vi "Communication.vi"(8 "Error In":errorcluster, 10 "Command":string, 11 "connection ID":refnum<k5>) -> (0 "Error Out":errorcluster, 2 "Data out":string, 3 "connection ID out":refnum<k5>)   [LabVIEW 2019, in "TCP2Foxconn.lvlib"]
uses:
  TCP2Foxconn.lvlib
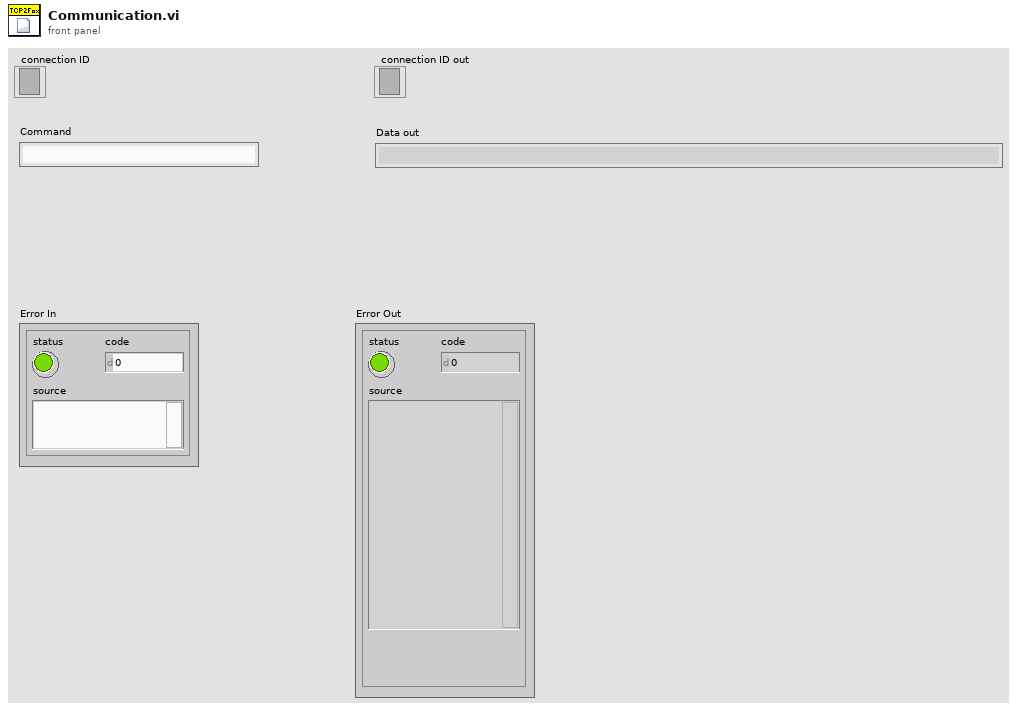
[diagram p1: front panel]
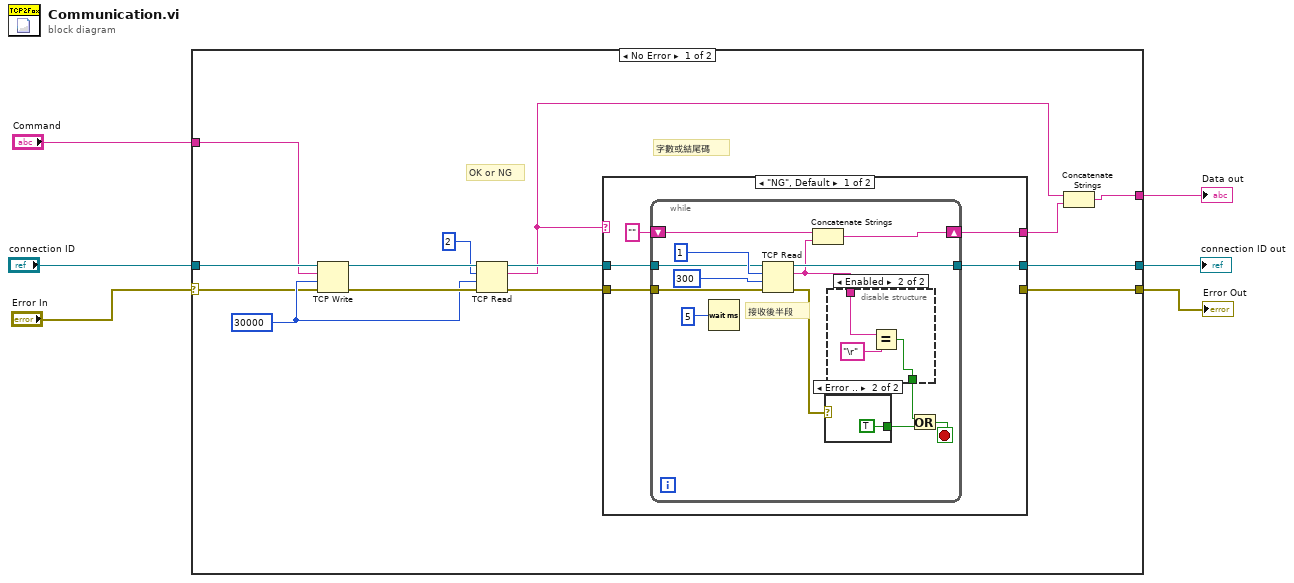
[diagram p0: block diagram]
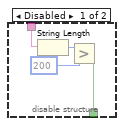
[diagram p2: hidden frame]
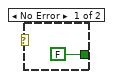
[diagram p3: hidden frame]
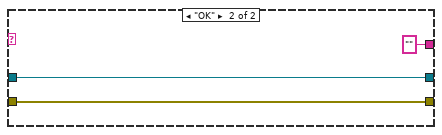
[diagram p4: hidden frame]
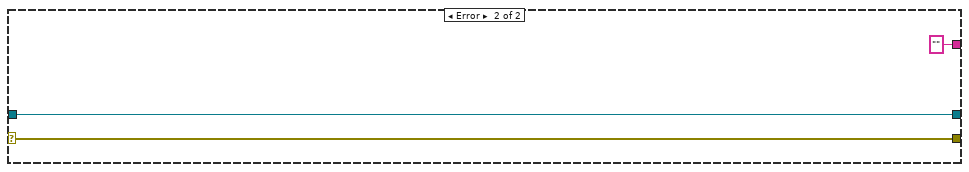
[diagram p5: hidden frame]
diagram:
  n1 = case shown="No Error" "Error In" {
    selector: "Error In" -> [w13 w52]
    tunnel: [w10 w52] -> w5
    tunnel: "connection ID" -> [w18 w53]
    tunnel: [w11 w53] -> w3
    tunnel: "Command" -> [w12 _]
    tunnel: [w7 "" ("data out")] -> w1
    frame No Error {
      w14 = 30000 ("timeout ms (25000)")
      # "字數或結尾碼"
      # "OK or NG"
      n2 = TCP Write(connection ID=w18, data in=w12, error in (no error)=w13, 9:w14) -> (connection ID out=w20:refnum<k5>, error out=w19:errorcluster)  [unwired: 1 out]
      n3 = TCP Read(connection ID=w20, bytes to read=2, error in (no error)=w19, 9:w14) -> (connection ID out=w15:refnum<k5>, data out=w9:string, error out=w16:errorcluster)  [unwired: 1 in]
      n4 = case shown="\"NG\", Default" w9 {
        tunnel: w16 -> [w24 w49]
        tunnel: w15 -> [w25 w50]
        tunnel: [_ w49] -> w10
        tunnel: [w22 w50] -> w11
        tunnel: [w21 ""] -> w8
        frame "NG", Default {
          n5 = while {
            tunnel: w25 -> [w36]
            tunnel: w24 -> [w35]
            tunnel: [w33] -> w22
            shift-right: [w30] -> w21
            shift-left: "" -> [w34]
            stop <- w29 stop-if-true
            # "接收後半段"
            n6 = Wait (ms)(milliseconds to wait=5) -> ()  [unwired: 1 out]
            n7 = TCP Read(connection ID=w36, bytes to read=1, error in (no error)=w35, 9:300 ("timeout ms (25000)")) -> (connection ID out=w33:refnum<k5>, data out=w26:string, error out=w32:errorcluster)  [unwired: 1 in]
            n8 = Concatenate Strings(w34, w26) -> (w30:string)
            n9 = case shown="Error .." w32 {
              tunnel: [FALSE TRUE] -> w27
              frame No Error {
              }
              frame Error {
              }
            }
            n10 = disable-structure shown="Enabled" {
              disable-tunnel: w26 -> [w42 w44]
              disable-tunnel: [w39 w43] -> w28
              frame Disabled {
                n11 = String Length(string=w42) -> (length=w41:i32)
                n12 = Greater?(x=w41, y=200) -> (0:w39:bool)
              }
              frame Enabled {
                n13 = Equal?(x=w44, y="\r") -> (x = y?=w43:bool)
              }
            }
            n14 = Or(x=w28, y=w27) -> (x .or. y?=w29:bool)
          }
        }
        frame "OK" {
        }
      }
      n15 = Concatenate Strings(w9, w8) -> (w7:string)
    }
    frame Error {
    }
  }
  "Error Out" <- w5
  "connection ID out" <- w3
  "Data out" <- w1
